vi "Poral Vector Vel From INS (SubVI).vi"(2 "Heading(deg)":dbl, 3 "Ve":dbl, 4 "Vn":dbl) -> (0 "Vy":dbl, 1 "Vx":dbl)   [LabVIEW 2015]
panel:
  # "Heading : INS에서 나온 헤딩 그대로 (deg.)\nVn : North Velocity (mps)\nVe : East Velocity (mps)\nVx : 차량 전방(x축) 속도(mps)\nVy : 차량 오른쪽 방향(y축) 속도(mps)\n\n극좌표계에서의 벡터 표현"
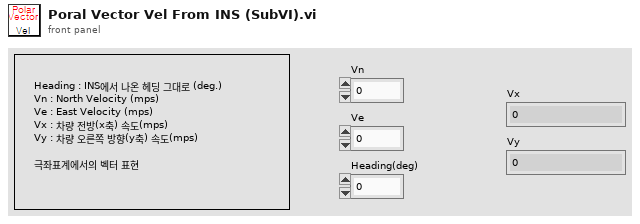
[diagram p1: front panel]
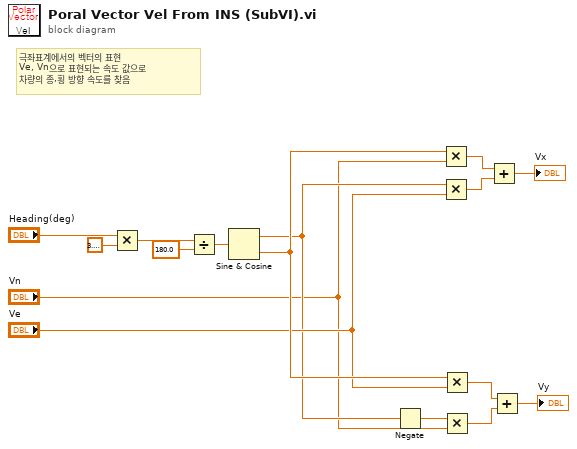
[diagram p0: block diagram]
diagram:
  # "극좌표계에서의 벡터의 표현\nVe, Vn으로 표현되는 속도 값으로\n차량의 종,횡 방향 속도를 찾음"
  n1 = Multiply(x="Heading(deg)", y=3.141592653589793) -> (x*y=w15:dbl)
  n2 = Divide(x=w15, y=180.0) -> (x/y=w12:dbl)
  n3 = Sine & Cosine(0:w12) -> (1:w4:dbl, 2:w6:dbl)
  n4 = Negate(x=w4) -> (-x=w9:dbl)
  n5 = Multiply(x=w6, y="Vn") -> (x*y=w8:dbl)
  n6 = Multiply(x=w4, y="Ve") -> (x*y=w7:dbl)
  n7 = Multiply(x=w6, y="Ve") -> (x*y=w2:dbl)
  n8 = Multiply(x=w9, y="Vn") -> (x*y=w1:dbl)
  n9 = Add(x=w8, y=w7) -> (x+y=→"Vx":dbl)
  n10 = Add(x=w2, y=w1) -> (x+y=→"Vy":dbl)
